vi "temp.vi"   [LabVIEW 2017]
uses:
  Error Handler/Controls/Error Data.ctl
  Error Handler/Controls/Error Type.ctl
types:
  T1 = typedef "Error Data.ctl" = cluster{"Error Type":T2, "Variant":variant}
  T2 = typedef "Error Type.ctl" = enum16{"Console Error", "Sensor Interface IO Error", "Process Step Error"}
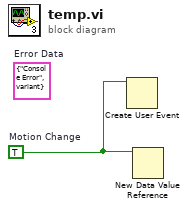
[diagram p0: block diagram]
diagram:
  w1 = TRUE  # Motion Change
  (unwired) T1 {"Error Type"=enum."Console Error", "Variant"=variant}  # Error Data
  n1 = Create User Event(user event datatype=w1) -> ()  [unwired: 1 in, 2 out]
  n2 = New Data Value Reference(data value=w1) -> ()  [unwired: 1 in, 2 out]
